vi "Select_actual_values.vi"(11 "CSMinfo in":T1 {"Окно с настройками"."Образец" items=["1", "2", "3"]; "Окно с настройками"."Условия окружающей среды" items=["Нормальная температура", "Максимальная температура", "Минимальная температура", "Вибрации типа А", "Вибрации типа Б"]; "Окно с настройками"."Напряжение источника" items=["12", "24"]; "Окно с настройками"."Режим звонка" items=["Автоматически (AT)", "Автоматически (реле)", "Вручную"]}) -> (0 "Условия окружающей среды":u16, 1 "Напряжение источника":u16, 2 "Образец":u16, 3 "Режим звонка":u16)   [LabVIEW 2018]
uses:
  CSMinfo.ctl
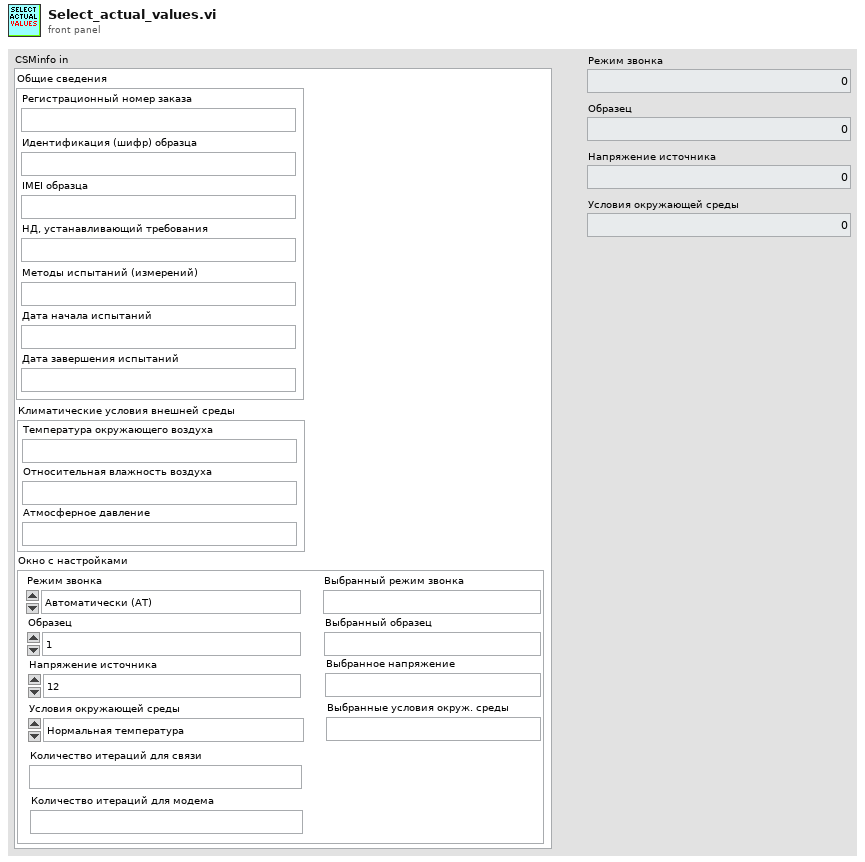
[diagram p1: front panel]
types:
  T1 = typedef "CSMinfo.ctl" = cluster{"Общие сведения":cluster{"Регистрационный номер заказа":string, "Идентификация (шифр) образца":string, "IMEI образца":string, "НД, устанавливающий требования":string, "Методы испытаний (измерений)":string, "Дата начала испытаний":string, "Дата завершения испытаний":string}, "Климатические условия внешней среды":cluster{"Температура окружающего воздуха":string, "Относительная влажность воздуха":string, "Атмосферное давление":string}, "Окно с настройками":cluster{"Режим звонка":u16, "Напряжение источника":u16, "Условия окружающей среды":u16, "Образец":u16, "Количество итераций для модема":string, "Количество итераций для связи":string, "Выбранный режим звонка":string, "Выбранный образец":string, "Выбранное напряжение":string, "Выбранные условия окруж. среды":string}}
  T2 = cluster{"Режим звонка":u16, "Напряжение источника":u16, "Условия окружающей среды":u16, "Образец":u16, "Количество итераций для модема":string, "Количество итераций для связи":string, "Выбранный режим звонка":string, "Выбранный образец":string, "Выбранное напряжение":string, "Выбранные условия окруж. среды":string}
  T3 = typedef "LVStringsAndValuesArrayTypeDef_U16.ctl" = cluster{"String":string, "Value":u16}[]
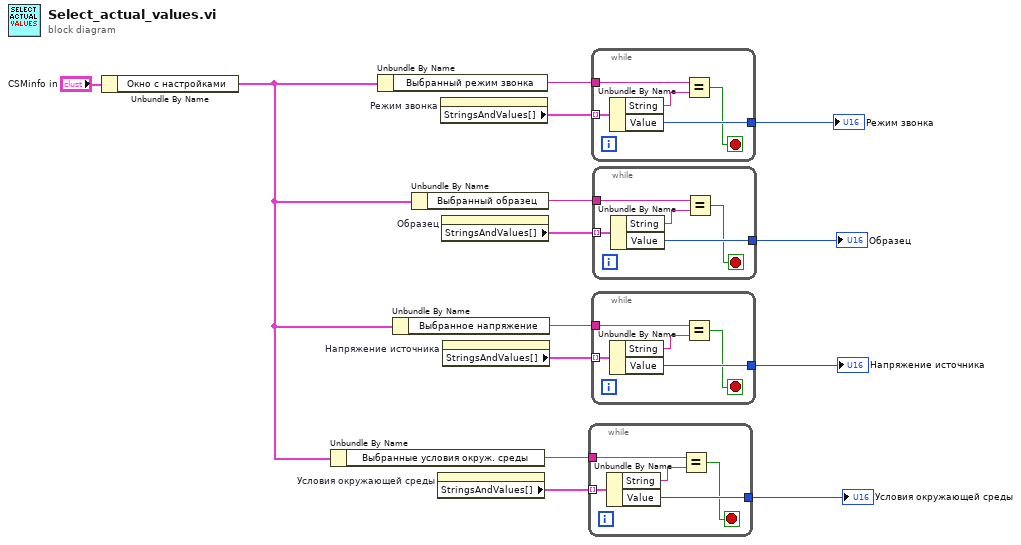
[diagram p0: block diagram]
diagram:
  n1 = Unbundle By Name("CSMinfo in") -> ("Окно с настройками"=w5:T2)
  n2 = Unbundle By Name(w5) -> ("Выбранные условия окруж. среды"=w8:string)
  n3 = Unbundle By Name(w5) -> ("Выбранный режим звонка"=w12:string)
  n4 = Unbundle By Name(w5) -> ("Выбранное напряжение"=w9:string)
  n5 = Unbundle By Name(w5) -> ("Выбранный образец"=w11:string)
  n6 = property on="Условия окружающей среды" class="Ring (strict)"() -> ("StringsAndValues[]"=w6:T3)  [unwired: 2 in, 2 out]
  n7 = property on="Режим звонка" class="Ring (strict)"() -> ("StringsAndValues[]"=w13:T3)  [unwired: 2 in, 2 out]
  n8 = property on="Образец" class="Ring (strict)"() -> ("StringsAndValues[]"=w10:T3)  [unwired: 2 in, 2 out]
  n9 = property on="Напряжение источника" class="Ring (strict)"() -> ("StringsAndValues[]"=w7:T3)  [unwired: 2 in, 2 out]
  n10 = while {
    tunnel: w6 -> [w19] mode=indexing
    tunnel: w8 -> [w18]
    tunnel: [w16] -> w1
    stop <- w15 stop-if-true
    n11 = Unbundle By Name(w19) -> ("String"=w17:string, "Value"=w16:u16)
    n12 = Equal?(x=w18, y=w17) -> (x = y?=w15:bool)
  }
  "Условия окружающей среды" <- w1
  n13 = while {
    tunnel: w13 -> [w24] mode=indexing
    tunnel: w12 -> [w23]
    tunnel: [w21] -> w4
    stop <- w20 stop-if-true
    n14 = Unbundle By Name(w24) -> ("String"=w22:string, "Value"=w21:u16)
    n15 = Equal?(x=w23, y=w22) -> (x = y?=w20:bool)
  }
  "Режим звонка" <- w4
  n16 = while {
    tunnel: w7 -> [w29] mode=indexing
    tunnel: w9 -> [w28]
    tunnel: [w26] -> w2
    stop <- w25 stop-if-true
    n17 = Unbundle By Name(w29) -> ("String"=w27:string, "Value"=w26:u16)
    n18 = Equal?(x=w28, y=w27) -> (x = y?=w25:bool)
  }
  "Напряжение источника" <- w2
  n19 = while {
    tunnel: w10 -> [w34] mode=indexing
    tunnel: w11 -> [w33]
    tunnel: [w31] -> w3
    stop <- w30 stop-if-true
    n20 = Unbundle By Name(w34) -> ("String"=w32:string, "Value"=w31:u16)
    n21 = Equal?(x=w33, y=w32) -> (x = y?=w30:bool)
  }
  "Образец" <- w3
